vi "RT TDMS controlled read.vi"(0 "start index":i64, 1 "tdms file":refnum<k34>, 2 "loop at EOF?":bool, 5 "Last Output":dbl, 7 "TDMS config":T1, 9 "Sample Size":i32, 11 "error in":errorcluster) -> (4 "next index":i64, 8 "new elements":dbl[](array[numeric]), 15 "error out":errorcluster)   [LabVIEW 2010, in "TDMS Custom Device.lvlib"]
uses:
  TDMS Custom Device.lvlib
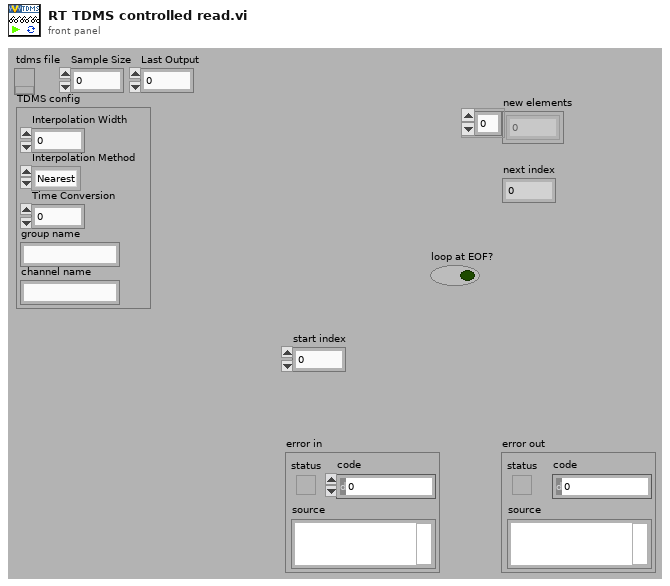
[diagram p1: front panel]
types:
  T1 = cluster{"Interpolation Width":i32, "Interpolation Method":enum16{"Nearest", "Linear", "Spline", "Cubic Hermite", "Lagrange", "Polynomial"}, "Time Conversion":dbl, "group name":string, "channel name":string}
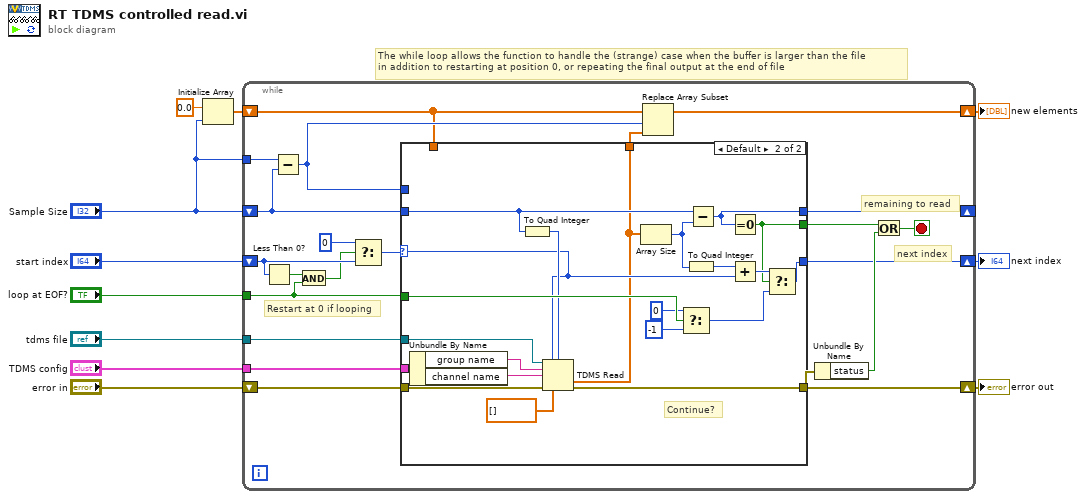
[diagram p0: block diagram]
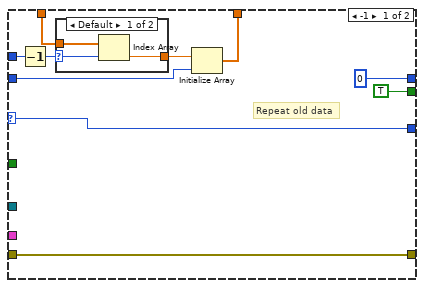
[diagram p2: hidden frame]
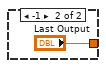
[diagram p3: hidden frame]
diagram:
  # "The while loop allows the function to handle the (strange) case when the buffer is larger than the file\nin addition to restarting at position 0, or repeating the final output at the end of file"
  n1 = Initialize Array(0.0 ("element"), "Sample Size") -> (w3:dbl[])
  n2 = while {
    shift-right: [w14] -> w9
    shift-left: w3 -> [w12]
    shift-right: [w32] -> _
    shift-left: "Sample Size" -> [w17]
    shift-right: [w27] -> w7
    shift-left: "start index" -> [w20]
    tunnel: "loop at EOF?" -> [w25]
    shift-right: [w24] -> w6
    shift-left: "error in" -> [w28]
    tunnel: "TDMS config" -> [w22]
    tunnel: "tdms file" -> [w21]
    tunnel: "Sample Size" -> [w15]
    stop <- w30 stop-if-true
    # "next index"
    # "remaining to read"
    # "Restart at 0 if looping"
    n3 = Less Than 0?(x=w20) -> (x < 0?=w26:bool)
    n4 = Subtract(x=w15, y=w17) -> (x-y=w13:i32)
    n5 = And(x=w26, y=w25) -> (x .and. y?=w18:bool)
    n6 = Select(t=i64 0 ("f"), s=w18, f=w20) -> (s? t:f=w23:i64)
    n7 = case shown="Default" w23 {
      selector: w23 -> [w40 w57]
      tunnel: [0 w67] -> w32
      tunnel: [TRUE w51] -> w31
      tunnel: w28 -> [w41 w66]
      tunnel: w17 -> [w33 w49]
      tunnel: [w40 w65] -> w27
      tunnel: w25 -> [_ w64]
      tunnel: [w41 w50] -> w24
      tunnel: w22 -> [_ w56]
      tunnel: w21 -> [_ w47]
      tunnel: [w35 w48] -> w16
      tunnel: w13 -> [w38 _]
      tunnel: w12 -> [w37 _]
      frame -1 {
        # "Repeat old data"
        n8 = Decrement(x=w38) -> (x-1=w36:i32)
        n9 = case shown="Default" w36 {
          selector: w36 -> [w44 _]
          tunnel: w37 -> [w45 _]
          tunnel: [w43 "Last Output"] -> w34
          frame Default {
            n10 = Index Array(array=w45, index=w44) -> (element=w43:dbl)
          }
          frame -1 {
          }
        }
        n11 = Initialize Array(w34, w33) -> (w35:dbl[])
      }
      frame Default {
        # "Continue?"
        n12 = Unbundle By Name(w56) -> ("group name"=w54:string, "channel name"=w55:string)
        n13 = To Quad Integer(1:w49) -> (0:w62:i64)
        n14 = TDMS Read(0:w47, 1:w57, 2:w62, 5:w54, 7:w55, 11:w66, 12:dbl[] []) -> (10:w48:dbl[], 15:w50:errorcluster)  [unwired: 4 out]
        n15 = Array Size(array=w48) -> (size(s)=w60:i32)
        n16 = Select(t=i64 0, s=w64, f=i64 -1) -> (s? t:f=w52:i64)
        n17 = To Quad Integer(1:w60) -> (0:w61:i64)
        n18 = Subtract(x=w49, y=w60) -> (x-y=w67:i32)
        n19 = Equal To 0?(x=w67) -> (x = 0?=w51:bool)
        n20 = Add(x=w61, y=w57) -> (x+y=w53:i64)
        n21 = Select(t=w53, s=w51, f=w52) -> (s? t:f=w65:i64)
      }
    }
    n22 = Replace Array Subset(array=w12, new element=w16, index=w13) -> (w14:dbl[])
    n23 = Unbundle By Name(w24) -> ("status"=w29:bool)
    n24 = Or(x=w31, y=w29) -> (x .or. y?=w30:bool)
  }
  "new elements" <- w9
  "next index" <- w7
  "error out" <- w6
